vi "Lockin_on_selection.vi"(9 "Cosine":waveform(dbl), 10 "Sine":waveform(dbl), 11 "Data":waveform(dbl)) -> (2 "Phase":dbl, 3 "Amplitude":dbl)   [LabVIEW 2015]
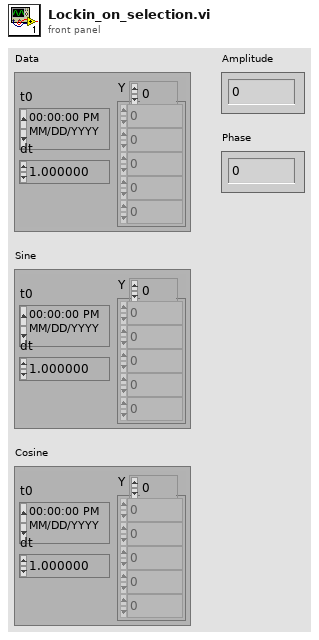
[diagram p1: front panel]
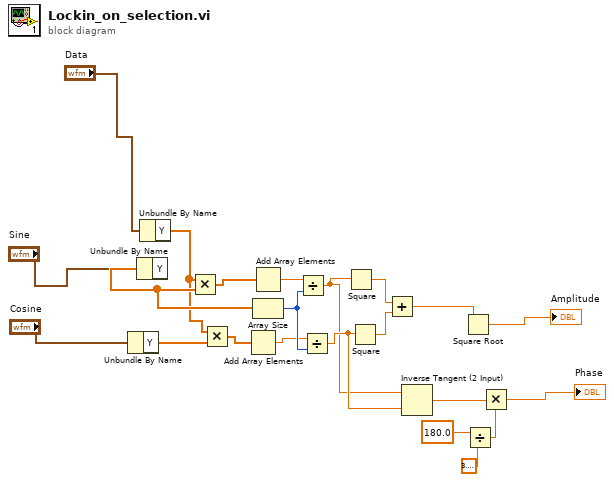
[diagram p0: block diagram]
diagram:
  n1 = Unbundle By Name("Cosine") -> ("Y"=w2:dbl[])
  n2 = Unbundle By Name("Sine") -> ("Y"=w6:dbl[])
  n3 = Unbundle By Name("Data") -> ("Y"=w1:dbl[])
  n4 = Multiply(x=w1, y=w6) -> (x*y=w4:dbl[])
  n5 = Multiply(x=w1, y=w2) -> (x*y=w5:dbl[])
  n6 = Add Array Elements(numeric array=w5) -> (sum=w8:dbl)
  n7 = Add Array Elements(numeric array=w4) -> (sum=w7:dbl)
  n8 = Array Size(array=w6) -> (size(s)=w9:i32)
  n9 = Divide(x=w7, y=w9) -> (x/y=w14:dbl)
  n10 = Divide(x=w8, y=w9) -> (x/y=w15:dbl)
  n11 = Square(x=w14) -> (x^2=w10:dbl)
  n12 = Square(x=w15) -> (x^2=w11:dbl)
  n13 = Add(x=w10, y=w11) -> (x+y=w12:dbl)
  n14 = Inverse Tangent (2 Input)(1:w15, 2:w14) -> (0:w19:dbl)
  n15 = Square Root(x=w12) -> (sqrt(x)=→"Amplitude":dbl)
  n16 = Divide(x=180.0, y=3.141592653589793) -> (x/y=w18:dbl)
  n17 = Multiply(x=w19, y=w18) -> (x*y=→"Phase":dbl)
